vi "led_cases.vi"() -> ()   [LabVIEW 2016]
uses:
  ledmatrix_default.ctl
  <vilib>/Instr/_visa.llb/VISA Configure Serial Port (Instr).vi
panel:
  in  "Numeric":dbl
  out "string":string
  in  "shift leds":bool
  in  "random leds":bool
  in  "Stuur data":bool
  in  "Clear leds":bool
  out "return count":u32
  in  "VISA resource name":refnum<visa-resource-name>="COM5"
  in  "stop":bool
  out "error out":errorcluster
  out "output array":u8[](array[numeric])
  out "String":string
  in  "Array":T1
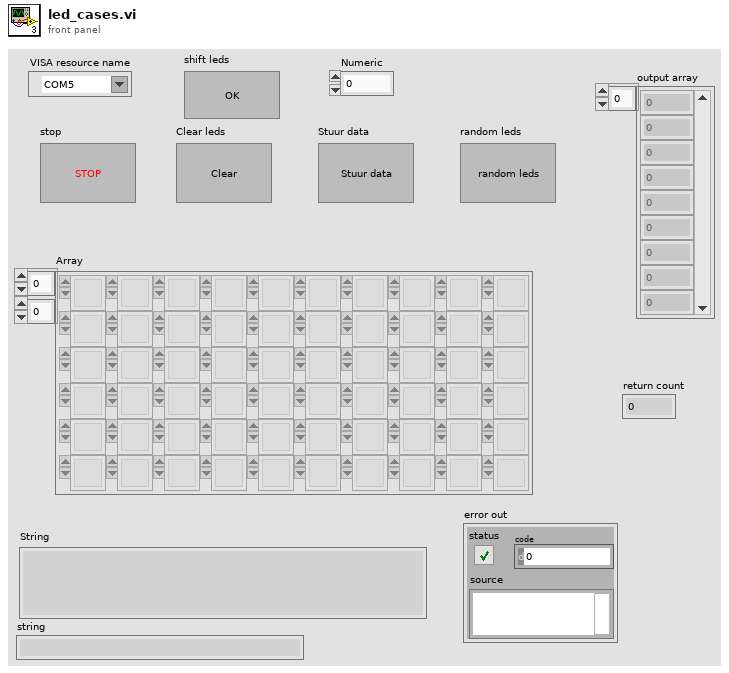
[diagram p1: front panel]
types:
  T1 = typedef "ledmatrix_default.ctl" = u8[][]
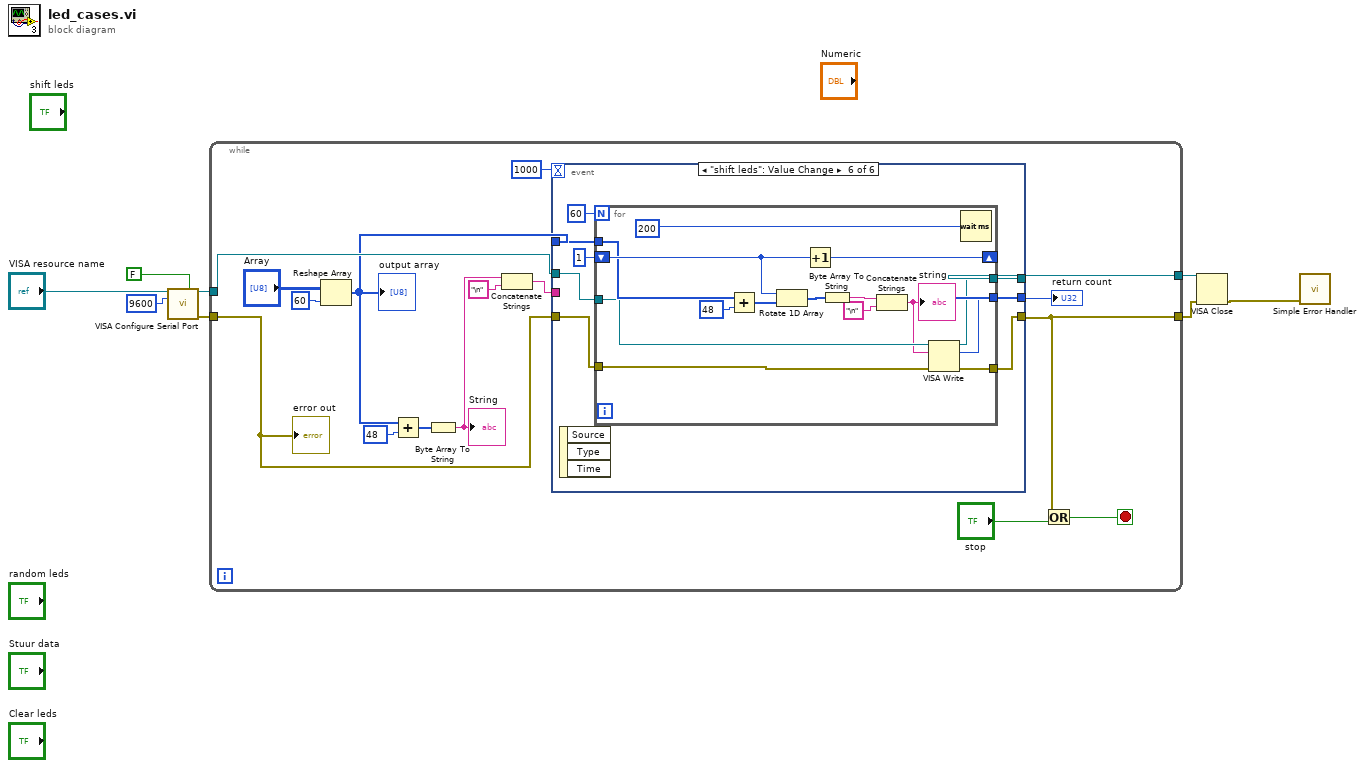
[diagram p0: block diagram]
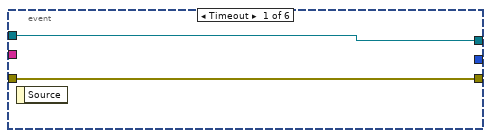
[diagram p2: hidden frame]
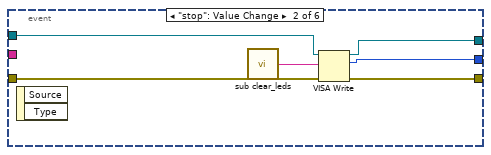
[diagram p3: hidden frame]
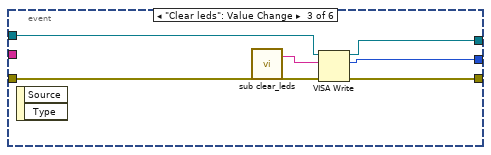
[diagram p4: hidden frame]
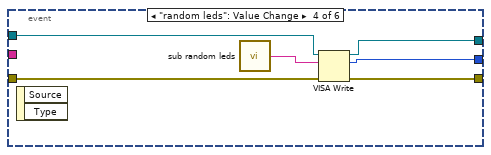
[diagram p5: hidden frame]
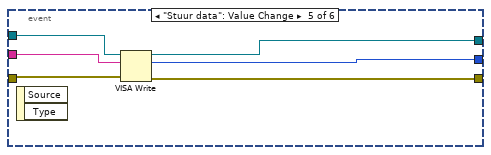
[diagram p6: hidden frame]
diagram:
  n1 = call-poly "VISA Configure Serial Port"("VISA resource name"="VISA resource name", "Enable Termination\nChar (T)"=FALSE ("Enable Termination\nChar (T)"), "baud rate (9600)"=u32 9600) -> ("VISA resource name out"=w6:refnum<visa-resource-name>, "error out"=w3:errorcluster)  [unwired: 11 in]
  n2 = while {
    tunnel: w6 -> [w18]
    tunnel: [w17] -> w2
    tunnel: [w14] -> w1
    tunnel: w3 -> [w10]
    stop <- w9 stop-if-true
    n3 = Reshape Array("Array", 60 ("dimension size")) -> (w11:u8[])
    "output array" <- w11
    n4 = Add(x=w11, y=u8 48 ("dimension size")) -> (x+y=w12:u8[])
    n5 = Byte Array To String(unsigned byte array=w12) -> (string=w22:string)
    "String" <- w22
    n6 = Concatenate Strings(w22, "\n" ("string")) -> (w15:string)
    n7 = event shown="[5] \"shift leds\": Value Change" {
      selector: _ -> [_ _ _ _ _ _]
      dyn-events: _ -> [_ _ _ _ _ _]
      timeout: 1000 -> [_ _ _ _ _ _]
      tunnel: w18 -> [w26 w32 w37 w44 w50 w56]
      tunnel: w10 -> [w25 w31 w36 w43 w49 w55]
      tunnel: [w26 w30 w34 w39 w48 w54] -> w17
      tunnel: [w25 w29 w35 w40 w47 w53] -> w14
      tunnel: w15 -> [_ _ _ _ w46 _]
      tunnel: [_ w28 w33 w41 w45 w52] -> w13
      tunnel: w11 -> [_ _ _ _ _ w57]
      event Timeout {
        n8 = event-data() -> ()  [unwired: 1 in, 1 out]
      }
      event "stop": Value Change {
        n9 = event-data() -> ()  [unwired: 1 in, 2 out]
        n10 = call "sub clear_leds.vi"() -> ("String"=w27:string)
        n11 = VISA Write(VISA resource name=w32, write buffer=w27, error in (no error)=w31) -> (VISA resource name out=w30:refnum<visa-resource-name>, return count=w28:u32, error out=w29:errorcluster)
      }
      event "Clear leds": Value Change {
        n12 = event-data() -> ()  [unwired: 1 in, 2 out]
        n13 = call "sub clear_leds.vi"() -> ("String"=w38:string)
        n14 = VISA Write(VISA resource name=w37, write buffer=w38, error in (no error)=w36) -> (VISA resource name out=w34:refnum<visa-resource-name>, return count=w33:u32, error out=w35:errorcluster)
      }
      event "random leds": Value Change {
        n15 = event-data() -> ()  [unwired: 1 in, 2 out]
        n16 = call "sub random leds.vi"() -> ("concatenated string"=w42:string)
        n17 = VISA Write(VISA resource name=w44, write buffer=w42, error in (no error)=w43) -> (VISA resource name out=w39:refnum<visa-resource-name>, return count=w41:u32, error out=w40:errorcluster)
      }
      event "Stuur data": Value Change {
        n18 = event-data() -> ()  [unwired: 1 in, 2 out]
        n19 = VISA Write(VISA resource name=w50, write buffer=w46, error in (no error)=w49) -> (VISA resource name out=w48:refnum<visa-resource-name>, return count=w45:u32, error out=w47:errorcluster)
      }
      event "shift leds": Value Change {
        n20 = event-data() -> ()  [unwired: 1 in, 3 out]
        n21 = for {
          N: 60 -> [_]
          shift-right: [w70] -> _
          shift-left: u8 1 -> [w71]
          tunnel: w57 -> [w65]
          tunnel: w56 -> [w64]
          tunnel: w55 -> [w63]
          tunnel: [w61] -> w54
          tunnel: [w60] -> w53
          tunnel: [w59] -> w52
          n22 = Add(x=w65, y=48) -> (x+y=w66:i32[])
          n23 = Rotate 1D Array(1:w66, 2:w71) -> (0:w72:i32[])
          n24 = Increment(x=w71) -> (x+1=w70:u8)
          n25 = Byte Array To String(unsigned byte array=w72) -> (string=w68:string)
          n26 = Concatenate Strings(w68, "\n") -> (w62:string)
          "string" <- w62
          n27 = VISA Write(VISA resource name=w64, write buffer=w62, error in (no error)=w63) -> (VISA resource name out=w61:refnum<visa-resource-name>, return count=w59:u32, error out=w60:errorcluster)
          n28 = Wait (ms)(milliseconds to wait=u32 200) -> ()  [unwired: 1 out]
        }
      }
    }
    "return count" <- w13
    n29 = Or(x=w14, y="stop") -> (x .or. y?=w9:bool)
    "error out" <- w10
  }
  n30 = VISA Close(VISA resource name=w2, error in (no error)=w1) -> (error out=w4:errorcluster)
  n31 = call <vilib>:"Simple Error Handler.vi"("error in (no error)"=w4) -> ()  [unwired: 4 in, 5 out]
